vi "Get ConfigType.vi"(8 "error in (no error)":errorcluster, 11 "Attribute.Config in":refnum<class "Attribute.Config.lvclass">) -> (0 "error out":errorcluster, 2 "Config Type":string, 3 "Attribute.Config out":refnum<class "Attribute.Config.lvclass">)   [LabVIEW 2013, in "Attribute.Config.lvclass"]
uses:
  Attribute.Config.lvclass
  Attribute.Config.lvclass/Attribute.Config.ctl
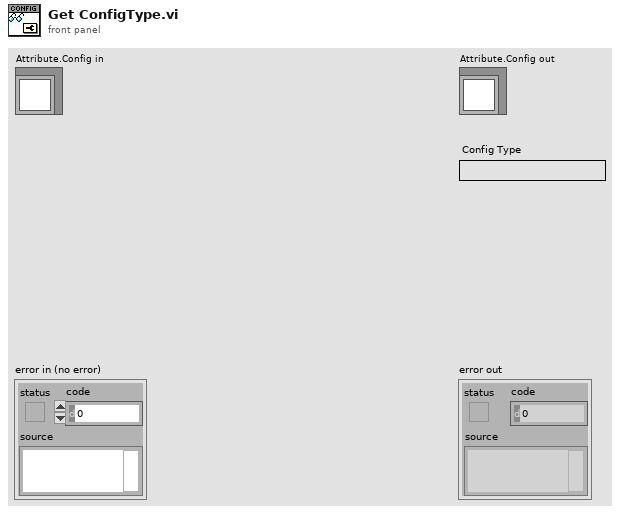
[diagram p1: front panel]
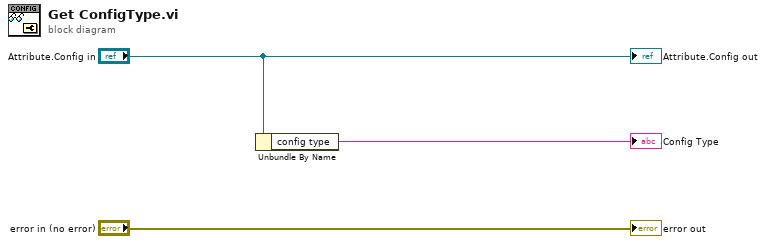
[diagram p0: block diagram]
diagram:
  n1 = Unbundle By Name("Attribute.Config in") -> ("config type"=→"Config Type":string)
  "error out" <- "error in (no error)"
  "Attribute.Config out" <- "Attribute.Config in"
